vi "计算旋转矩形-找一字槽单边.vi"(6 "矩形":cluster{"X":dbl, "Y":dbl}, 8 "旋转角度":dbl, 10 "矩形中心":cluster{dbl, dbl}, 11 "Img输入":T1) -> (2 "ROI Descriptor":T2 {"Contours"."Type" items=["No Selection", "Point", "Line", "Rectangle", "Oval", "Polygon", "Freehand Region", "Annulus", "Unused2", "Unused3", "Broken Line", "Freehand Line", "Rotated Rectangle"]}, 3 "Image Out":T1)   [LabVIEW 2014]
uses:
  <vilib>/vision/Image Controls.llb/IMAQ Image.ctl
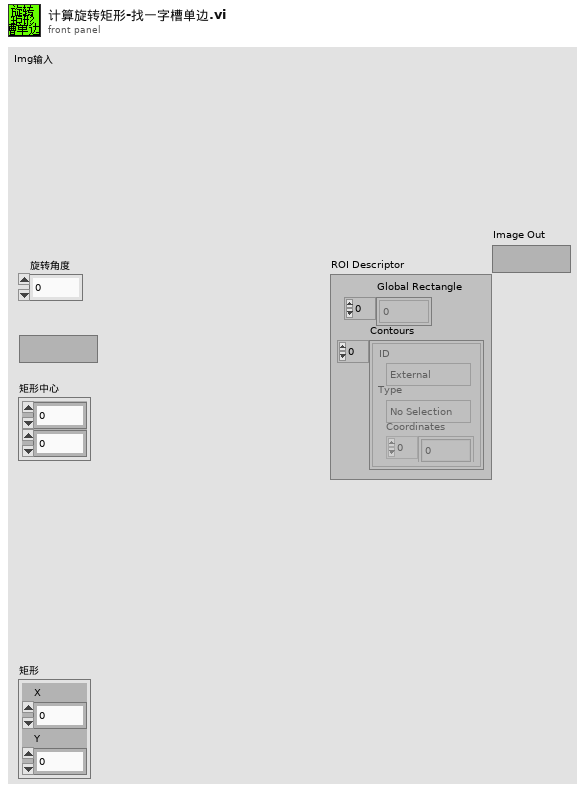
[diagram p1: front panel]
types:
  T1 = typedef "IMAQ Image.ctl" = refnum<image>
  T2 = typedef "ROI Descriptor" = cluster{"Global Rectangle":i32[], "Contours":cluster{"ID":enum32{"External", "Internal"}, "Type":u32, "Coordinates":i32[]}[]}
  T3 = typedef "IMAQ Rectangle" = cluster{"Left":i32, "Top":i32, "Right":i32, "Bottom":i32, "Rotation":dbl}
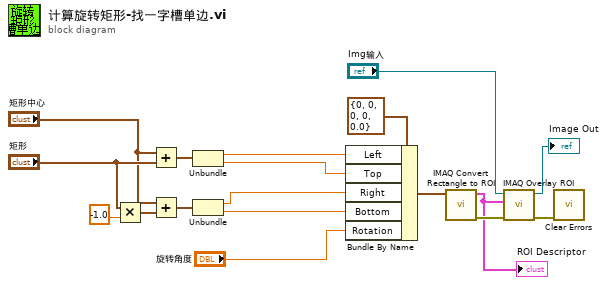
[diagram p0: block diagram]
diagram:
  n1 = Multiply(x="矩形", y=-1.0) -> (x*y=w16:cluster{"X":dbl, "Y":dbl})
  n2 = Add(x="矩形中心", y="矩形") -> (x+y=w11:cluster{dbl, dbl})
  n3 = Add(x="矩形中心", y=w16) -> (x+y=w10:cluster{dbl, dbl})
  n4 = Unbundle(w11) -> (w9:dbl, w8:dbl)
  n5 = Unbundle(w10) -> (w7:dbl, w6:dbl)
  n6 = Bundle By Name(cluster=T3 {"Left"=0, "Top"=0, "Right"=0, "Bottom"=0, "Rotation"=0.0} ("Rectangle输入"), "Left"=w9, "Top"=w8, "Right"=w7, "Bottom"=w6, "Rotation"="旋转角度") -> (w5:T3)
  n7 = call "IMAQ Convert Rectangle to ROI"("Rectangle"=w5) -> ("error out"=w4:errorcluster, "ROI Descriptor"=w2:T2)  [unwired: 8 in]
  "ROI Descriptor" <- w2
  n8 = call "IMAQ Overlay ROI"("error in (no error)"=w4, "ROI Descriptor"=w2, "Image"="Img输入") -> ("error out"=w3:errorcluster, "Image Out"=→"Image Out":T1)  [unwired: 7 in]
  n9 = call <vilib>:"Clear Errors.vi"("error in (no error)"=w3) -> ()  [unwired: 5 in, 2 out]
